vi "Callback Change Channel Type.vi"(6 "Variant":variant, 8 "error in (no error)":errorcluster, 9 "Old Values":string[][](array[string]), 10 "object ref in":T2, 11 "Table Change":T3) -> (0 "error out":errorcluster)   [LabVIEW 2014, in "Daqmx Module editor node.lvclass"]
doc: "This VI gets called automatically when changes are made to the 'Channel Direction' column of the table and must handle changes appropriately. Register this callback using the appropriate 'Define Column' VI from the Table API."
uses:
  Daqmx Module editor node.lvclass
  <vilib>/NI/DCAF/Tag Editor Core/Table API/Table Manager/Cell Change.ctl
  <vilib>/NI/DCAF/Tag Editor Core/Table API/Table Manager/object ref.ctl
  <vilib>/NI/DCAF/Tag Editor Core/Configuration Editor/Classes/Engine Parent/Engine Parent Editor Node.lvclass
  <vilib>/NI/DCAF/Tag Editor Core/Configuration Editor/Classes/Module editor node/module editor node.lvclass
  module/configuration/Channel Type.ctl
  module/configuration/Daqmx Module configuration.lvclass
  module/configuration/Daqmx Module configuration.lvclass/Daqmx Module configuration.ctl
  module/configuration/Get Line Name.vi
  <vilib>/NI/Tag Bus Module Framework/module configuration/FindDuplicate.vi
  <vilib>/Utility/error.llb/Error Cluster From Error Code.vi
  <vilib>/NI/Tag Bus Module Framework/channel/TBM channel.lvclass
  <vilib>/NI/DCAF/Tag Editor Core/Table API/Table Manager.lvlib
  <vilib>/NI/DCAF/Tag Editor Core/Table API/Table Manager/Table Manager.lvclass
panel:
  in  "Channel Type":T1
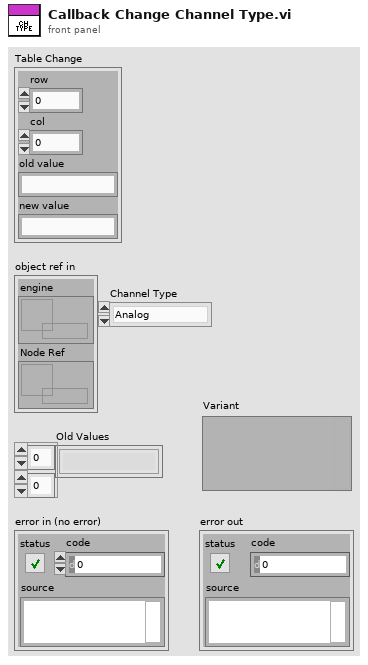
[diagram p1: front panel]
types:
  T1 = typedef "Daqmx Module configuration.lvclass/Channel Type.ctl" = enum16{"Analog", "Digital"}
  T2 = typedef "Table Manager.lvlib/Table Manager.lvclass/object ref.ctl" = cluster{"engine":refnum<data-value>, "Node Ref":refnum<data-value>}
  T3 = typedef "Table Manager.lvlib/Cell Change.ctl" = cluster{"row":i32, "col":i32, "old value":string, "new value":string}
  T4 = typedef "Daqmx Module configuration.lvclass/Line.ctl" = cluster{"channel":refnum<class "TBM channel.lvclass">, "Physical Channel":string, "Channel Type":T1, "Parameters":variant}
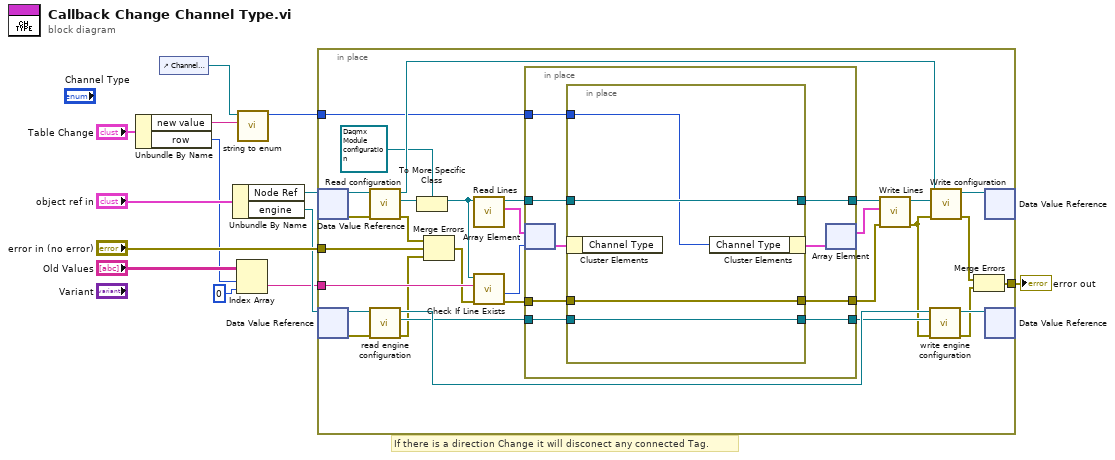
[diagram p0: block diagram]
diagram:
  # "If there is a direction Change it will disconect any connected Tag."
  n1 = Unbundle By Name("Table Change") -> ("new value"=w3:string, "row"=w4:i32)
  n2 = control-ref of="Channel Type"() -> (w1:refnum<vi>)
  n3 = Unbundle By Name("object ref in") -> ("Node Ref"=w10:refnum<data-value>, "engine"=w9:refnum<data-value>)
  n4 = Index Array(array="Old Values", index (row)=w4, index (col)=0 ("disabled index (col)")) -> (element=w5:string)
  n5 = call <vilib>:"string to enum.vi"("String"=w3, "Enum"=w1) -> ("Value"=w2:i32)  [unwired: 8 in, 1 out]
  n6 = in-place {
    in-place-border: [w37] -> w13
    in-place-border: "error in (no error)" -> [w15]
    in-place-border: w2 -> [w25]
    in-place-border: w5 -> [w24]
    n7 = in-place-dvr #1(w10) -> (w34:refnum<class "module editor node.lvclass">, w36:errorcluster)
    n8 = in-place-dvr #2(w9) -> (w43:refnum<class "Engine Parent Editor Node.lvclass">, w44:errorcluster)
    n9 = call-dynamic "Read configuration.vi"("error in"=w36, "NISE_CEF_serializable node in"=w34) -> ("error out"=w35:errorcluster, "configuration"=w32:refnum<class "NISE_CEF_serializable configuration.lvclass">, "NISE_CEF_serializable node out"=w33:refnum<class "module editor node.lvclass">)  [unwired: 7 in]
    n10 = call <vilib>:"read engine configuration.vi"("error in"=w44, "Engine Parent Editor Node in"=w43) -> ("error out"=w14:errorcluster, "engine configuration"=w21:refnum<class "engine configuration.lvclass">, "Engine Parent Editor Node out"=w40:refnum<class "Engine Parent Editor Node.lvclass">)  [unwired: 7 in]
    n11 = To More Specific Class(target class=refnum<class "Daqmx Module configuration.lvclass"> refnum ("tag bus configurable plugin module configuration"), reference=w32) -> (specific class reference=w29:refnum<class "Daqmx Module configuration.lvclass">)  [unwired: 1 in, 1 out]
    n12 = Merge Errors(w35, w15, w14) -> (w19:errorcluster)
    n13 = call "Read Lines.vi"("Daqmx Module configuration in"=w29) -> ("Lines"=w28:T4[], "Daqmx Module configuration out"=w23:refnum<class "Daqmx Module configuration.lvclass">)  [unwired: 8 in, 1 out]
    n14 = call-dynamic "Check If Line Exists.vi"("error in"=w19, "Name to Locate"=w24, "Daqmx Module configuration in"=w29) -> ("error out"=w18:errorcluster, "Index"=w26:i32)  [unwired: 4 in, 3 out]
    n15 = in-place {
      in-place-border: w25 -> [w51]
      in-place-border: w23 -> [w50]
      in-place-border: [w49] -> w22
      in-place-border: w21 -> [w48]
      in-place-border: [w47] -> w20
      in-place-border: w18 -> [w46]
      in-place-border: [w45] -> w17
      n16 = in-place-array #3(w28, w26) -> (w53:T4)
      n17 = in-place {
        in-place-border: w51 -> [w55]
        in-place-border: w50 -> [w57]
        in-place-border: [w57] -> w49
        in-place-border: w48 -> [w56]
        in-place-border: [w56] -> w47
        in-place-border: w46 -> [w54]
        in-place-border: [w54] -> w45
        n18 = in-place-cluster #4(w53) -> ()  [unwired: 1 out]
        n19 = in-place-cluster #4("Channel Type"=w55) -> (w52:T4)
      }
      n20 = in-place-array #3(w52) -> (w27:T4[])  [unwired: 1 out]
    }
    n21 = call "Write Lines.vi"("error in (no error)"=w17, "Lines"=w27, "Daqmx Module configuration in"=w22) -> ("error out"=w16:errorcluster, "Daqmx Module configuration out"=w30:refnum<class "Daqmx Module configuration.lvclass">)  [unwired: 7 in]
    n22 = call <vilib>:"write engine configuration.vi"("error in"=w16, "engine configuration"=w20, "Engine Parent Editor Node in"=w40) -> ("error out"=w39:errorcluster, "Engine Parent Editor Node out"=w42:refnum<class "Engine Parent Editor Node.lvclass">)  [unwired: 7 in]
    n23 = call-dynamic "Write configuration.vi"("error in"=w16, "configuration"=w30, "NISE_CEF_serializable node in"=w33) -> ("error out"=w38:errorcluster, "NISE_CEF_serializable node out"=w41:refnum<class "module editor node.lvclass">)  [unwired: 7 in]
    n24 = Merge Errors(w38, w39) -> (w37:errorcluster)
    n25 = in-place-dvr #1(w41) -> ()  [unwired: 2 out]
    n26 = in-place-dvr #2(w42) -> ()  [unwired: 2 out]
  }
  "error out" <- w13
